vi "SetActiveDevs.vi"(6 "Legacy (f)?":bool, 8 "error in (no error)":errorcluster, 10 "Device DAQmx Names":string[](array[string])) -> (0 "error out":errorcluster)   [LabVIEW 2011]
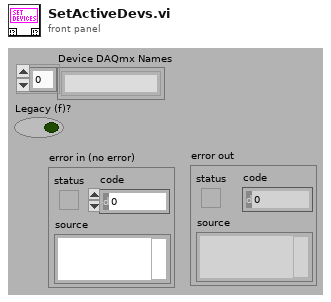
[diagram p1: front panel]
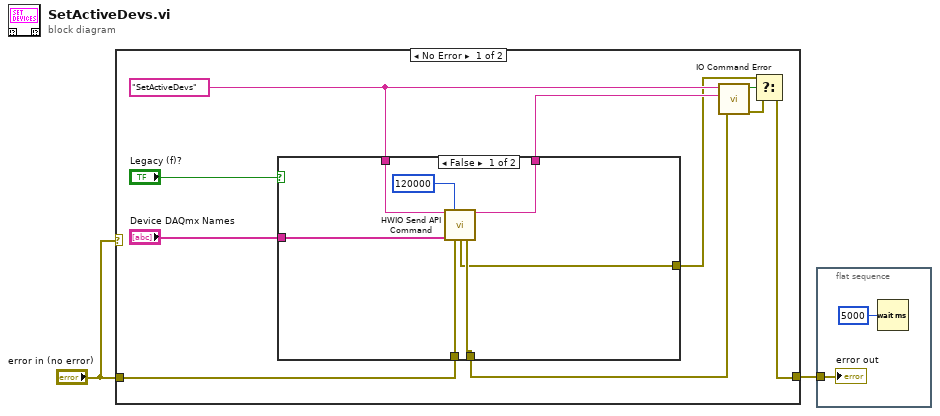
[diagram p0: block diagram]
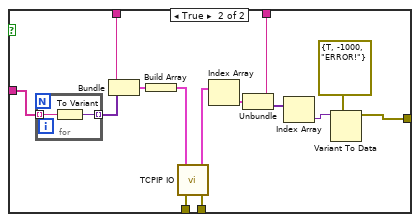
[diagram p2: hidden frame]
diagram:
  n1 = case shown="No Error" "error in (no error)" {
    tunnel: "error in (no error)" -> [w12 w36]
    tunnel: [w6 w36] -> w2
    frame No Error {
      w10 = "SetActiveDevs"
      n2 = case shown="False" "Legacy (f)?" {
        tunnel: w12 -> [w19 w33]
        tunnel: [w15 w31] -> w11
        tunnel: w10 -> [w18 w30]
        tunnel: [w17 w29] -> w9
        tunnel: "Device DAQmx Names" -> [w16 w21]
        tunnel: [w14 w20] -> w4
        frame False {
          n3 = call "HWIO Send API Command.vi"("Action"=w18, "Timeout ms (5000)"=120000, "String"=w16, "error in (no error)"=w19) -> ("Action out"=w17:string, "HWError"=w14:errorcluster, "error out"=w15:errorcluster)  [unwired: 4 in, 5 out]
        }
        frame True {
          n4 = for {
            tunnel: [w35] -> w22 mode=indexing
            tunnel: w21 -> [w34] mode=indexing
            n5 = To Variant(anything=w34) -> (Variant=w35:variant)
          }
          n6 = Bundle(w30, w22) -> (w32:cluster{string, variant[]})  [unwired: 1 out]
          n7 = Build Array(w32) -> (w28:cluster{string, variant[]}[])
          n8 = call "TCPIP IO.vi"("error in (no error)"=w33, "Commands"=w28) -> ("error out"=w31:errorcluster, "Responses"=w26:cluster{string, variant[]}[])  [unwired: 1 in, 3 out]
          n9 = Index Array(array=w26) -> (element=w27:cluster{string, variant[]})  [unwired: 1 in]
          n10 = Unbundle(w27) -> (w29:string, w25:variant[])
          n11 = Index Array(array=w25) -> (element=w24:variant)  [unwired: 1 in]
          n12 = Variant To Data(type=errorcluster {"status"=TRUE, "code"=-1000, "source"="ERROR!"} ("error out"), Variant=w24) -> (data=w20:errorcluster)  [unwired: 1 in, 1 out]
        }
      }
      n13 = call "IO Command Error.vi"("error in (no error)"=w11, "Command Returned (\"\")"=w9, "Command Sent (\"\")"=w10) -> ("error out"=w7:errorcluster, "HW ERR?"=w8:bool)  [unwired: 3 out]
      n14 = Select(t=w4, s=w8, f=w7) -> (s? t:f=w6:errorcluster)
    }
    frame Error {
    }
  }
  n15 = flat-sequence {
    tunnel: w2 -> [w38]
    frame #0 {
      n16 = Wait (ms)(milliseconds to wait=u32 5000) -> ()  [unwired: 1 out]
      "error out" <- w38
    }
  }
